vi "_rsscope Get Trace Data.vi"(4 "Force ASCII (F)":bool, 6 "Wait for OPC (F)":bool, 8 "error in (no error)":errorcluster, 10 "Command":string, 11 "VISA resource name":refnum<visa-resource-name>) -> (0 "error out":errorcluster, 1 "Values":dbl[](array[numeric]) format="%.2e", 3 "VISA resource name out":refnum<visa-resource-name>)   [LabVIEW 2014]
doc: "This VI returns the instrument's trace as double array."
uses:
  rsidr_core.llb/rsscope_rsidr_core.lvlib
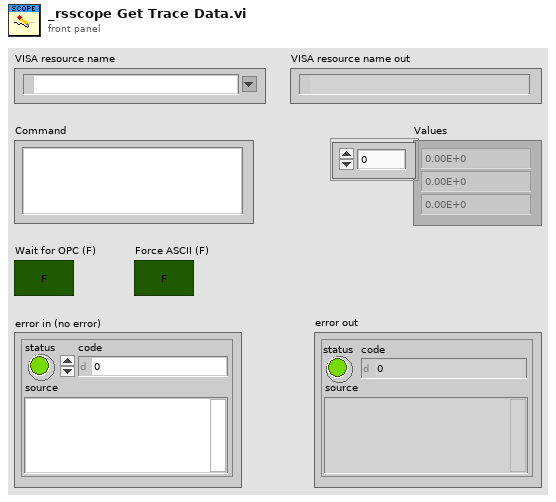
[diagram p1: front panel]
types:
  T1 = typedef "rsscope_rsidr_core.lvlib/type_Session_Data.ctl" = cluster{"IDN string":string, "Instrument FW":string, "Instr type":string, "Instr type for err. msg.":string, "Installed Options":string[], "Ignore Error Messages":string, "Logging params":variant, "OPC Timeout":i32, "VISA Timeout":i32, "STB Poll VISA Timeout":i32, "Additional Flags":i32, "Wait Before Read":i32, "Wait Before Write":i32, "Option String Flags":i32, "IO Segment Size":i64, "VISA Access Mode":T2, "Interface Type":T3, "OPC Wait Mode":T4, "Bin Float Number  Format":T5, "Bin Integer Number Format":T6, "Simulate":bool, "VXIcapable":bool, "Duplicate Session":bool, "Add LF to Write":bool, "Logging":bool, "Fast Sweep":bool, "Query Instrument Status":bool, "Check Range":bool, "Check Options":bool}
  T2 = typedef "rsscope_rsidr_core.lvlib/type_VisaAccessMode.ctl" = u16
  T3 = typedef "rsscope_rsidr_core.lvlib/type_InterfaceType.ctl" = enum16{"Unknown", "GPIB", "VXI", "GPIB_VXI", "ASRL", "PXI", "TCPIP", "USB", "SOCKET"}
  T4 = typedef "rsscope_rsidr_core.lvlib/type_OPC_Wait_Mode.ctl" = enum16{"STBpolling", "STBpollingSlow", "STBpollingSuperSlow", "ServiceRequest", "OPCquery"}
  T5 = typedef "rsscope_rsidr_core.lvlib/type_Binary_Float_Number_Format.ctl" = enum16{"Float_4_Bytes_Swapped", "Float_4_Bytes", "Double_8_Bytes_Swapped", "Double_8_Bytes"}
  T6 = typedef "rsscope_rsidr_core.lvlib/type_Binary_Integer_Number_Format.ctl" = enum16{"Int32_4_Bytes_Swapped", "Int32_4 Bytes", "Int16_2_Bytes_Swapped", "Int16_2_Bytes"}
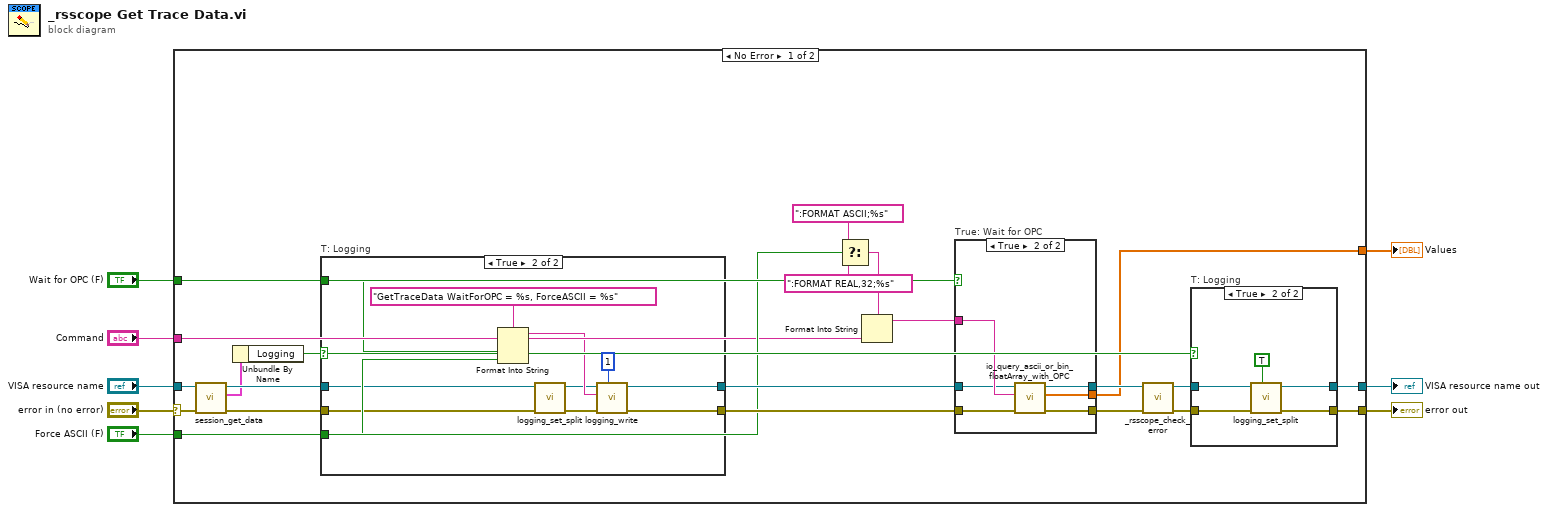
[diagram p0: block diagram]
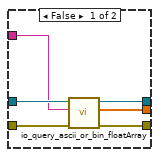
[diagram p2: hidden frame]
diagram:
  n1 = case shown="No Error" "error in (no error)" {
    selector: "error in (no error)" -> [w30 w64]
    tunnel: "Command" -> [w10 _]
    tunnel: "Wait for OPC (F)" -> [w12 _]
    tunnel: "Force ASCII (F)" -> [w11 _]
    tunnel: "VISA resource name" -> [w29 w63]
    tunnel: [w22 w64] -> w3
    tunnel: [w21 w63] -> w2
    tunnel: [w9 _] -> w1
    frame No Error {
      n2 = call "session_get_data.vi"("error in"=w30, "VISA resource name"=w29) -> ("error out"=w28:errorcluster, "Session User Data out"=w23:T1, "VISA resource name out"=w27:refnum<visa-resource-name>)  [unwired: 6 in, 1 out]
      n3 = Unbundle By Name(w23) -> ("Logging"=w24:bool)
      n4 = case "T: Logging" shown="True" w24 {
        tunnel: w28 -> [w51 w57]
        tunnel: [w51 w53] -> w16
        tunnel: w27 -> [w50 w56]
        tunnel: [w50 w52] -> w15
        tunnel: w12 -> [_ w59]
        tunnel: w11 -> [_ w58]
        frame False {
        }
        frame True {
          n5 = Format Into String(format string="GetTraceData WaitForOPC = %s, ForceASCII = %s", w59, w58) -> (resulting string=w62:string)  [unwired: 2 in, 1 out]
          n6 = call "logging_set_split.vi"("error in"=w57, "VISA resource name"=w56) -> ("error out"=w55:errorcluster, "VISA resource name out"=w54:refnum<visa-resource-name>)  [unwired: 8 in]
          n7 = call "logging_write.vi"("Add call chain offset\n(No call chain)"=1 ("Add call chain offset\n(No call chain)"), "error in"=w55, "String to write"=w62, "VISA resource name"=w54) -> ("error out"=w53:errorcluster, "VISA resource name out"=w52:refnum<visa-resource-name>)  [unwired: 6 in]
        }
      }
      n8 = Select(t=":FORMAT ASCII;%s", s=w11, f=":FORMAT REAL,32;%s") -> (s? t:f=w17:string)
      n9 = Format Into String(format string=w17, w10) -> (resulting string=w20:string)  [unwired: 2 in, 1 out]
      n10 = case "True: Wait for OPC" shown="True" w12 {
        tunnel: w16 -> [w36 w40]
        tunnel: w15 -> [w35 w39]
        tunnel: [w34 w38] -> w14
        tunnel: [w33 w37] -> w13
        tunnel: w20 -> [w32 w42]
        tunnel: [w31 w41] -> w9
        frame False {
          n11 = call "io_query_ascii_or_bin_floatArray.vi"("error in"=w36, "Query"=w32, "VISA resource name"=w35) -> ("error out"=w34:errorcluster, "Numbers out"=w31:dbl[], "VISA resource name out"=w33:refnum<visa-resource-name>)  [unwired: 5 in, 1 out]
        }
        frame True {
          n12 = call "io_query_ascii_or_bin_floatArray_with_OPC.vi"("error in"=w40, "Query"=w42, "VISA resource name"=w39) -> ("error out"=w38:errorcluster, "Numbers out"=w41:dbl[], "VISA resource name out"=w37:refnum<visa-resource-name>)  [unwired: 5 in, 1 out]
        }
      }
      n13 = call "_rsscope_check_error.vi"("error in (no error)"=w14, "VISA resource name"=w13) -> ("error out"=w25:errorcluster, "VISA resource name out"=w26:refnum<visa-resource-name>)  [unwired: 8 in]
      n14 = case "T: Logging" shown="True" w24 {
        tunnel: w25 -> [w44 w49]
        tunnel: [w44 w47] -> w22
        tunnel: w26 -> [w43 w48]
        tunnel: [w43 w46] -> w21
        frame False {
        }
        frame True {
          n15 = call "logging_set_split.vi"("Evaluate section error (F)"=TRUE, "error in"=w49, "VISA resource name"=w48) -> ("error out"=w47:errorcluster, "VISA resource name out"=w46:refnum<visa-resource-name>)  [unwired: 7 in]
        }
      }
    }
    frame Error {
    }
  }
  "error out" <- w3
  "VISA resource name out" <- w2
  "Values" <- w1
